vi "Get IC.vi"(8 "error in (no error)":errorcluster, 10 "Domain":refnum<class "NI_Domain.lvclass">, 11 "IC_2D_VIRef in":refnum<class "NI_IC_2D_VIRef.lvclass">) -> (0 "error out":errorcluster, 2 "IC":variant, 3 "IC_2D_VIRef out":refnum<class "NI_IC_2D_VIRef.lvclass">)   [LabVIEW 2020, in "NI_PDE.lvlib" / "NI_IC_2D_VIRef.lvclass"]
uses:
  <vilib>/gmath/pde.llb/ICClass/IC_2D_VIRef/NI_IC_2D_VIRef.lvclass
  <vilib>/gmath/pde.llb/DomainClass/NI_Domain.lvclass
  <vilib>/gmath/pde.llb/ICClass/IC_2D_VIRef/IC Data.ctl
  <vilib>/gmath/pde.llb/Common/PDE_IC Type.ctl
  <vilib>/gmath/pde.llb/ICClass/IC_2D_VIRef/NI_IC_2D_VIRef.lvclass/NI_IC_2D_VIRef.ctl
  <vilib>/gmath/NI_PDE.lvlib
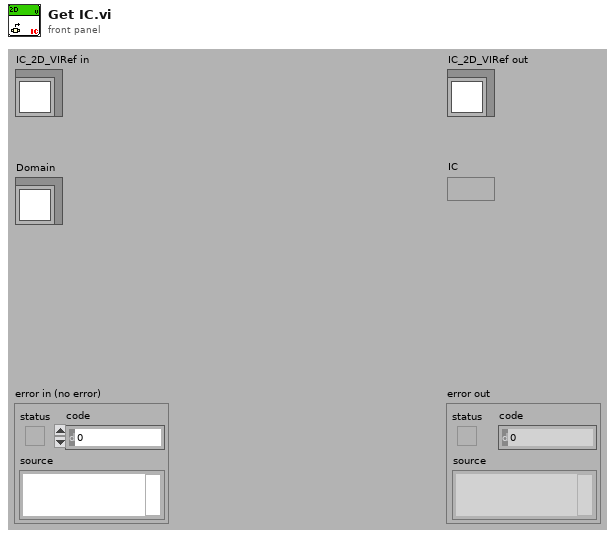
[diagram p1: front panel]
types:
  T1 = typedef "NI_PDE.lvlib/NI_IC_2D_VIRef.lvclass/IC Data.ctl" = cluster{"type":T2, "H":refnum<vi>, "data":variant}
  T2 = typedef "NI_PDE.lvlib/PDE_IC Type.ctl" = i32
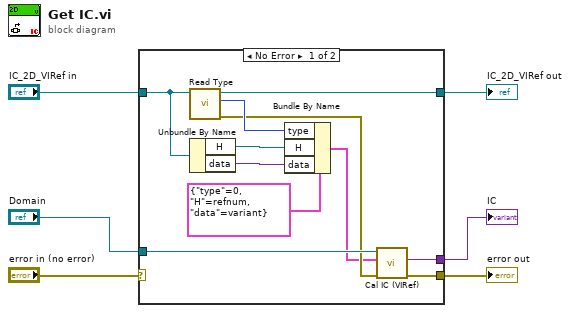
[diagram p0: block diagram]
diagram:
  n1 = case shown="No Error" "error in (no error)" {
    selector: "error in (no error)" -> [_ w19]
    tunnel: [w17 w18] -> w6
    tunnel: "IC_2D_VIRef in" -> [w14 w18]
    tunnel: "Domain" -> [w11 _]
    tunnel: [w7 w19] -> w3
    tunnel: [w8 _] -> w2
    frame No Error {
      n2 = call-dynamic "Read Type.vi"("IC.lvclass in"=w14) -> ("error out"=w10:errorcluster, "IC type"=w15:T2, "IC.lvclass out"=w17:refnum<class "NI_IC_2D_VIRef.lvclass">)  [unwired: 1 in, 7 out]
      n3 = Unbundle By Name(w14) -> ("H"=w13:refnum<vi>, "data"=w12:variant)
      n4 = Bundle By Name(cluster=T1 {"type"=0, "H"=refnum, "data"=variant} ("IC data"), "type"=w15, "H"=w13, "data"=w12) -> (w9:T1)
      n5 = call-dynamic "Cal IC (VIRef).vi"("error in (no error)"=w10, "IC in"=w9, "Domain in"=w11) -> ("error out"=w7:errorcluster, "IC out"=w8:variant)  [unwired: 7 out]
    }
    frame Error {
    }
  }
  "IC" <- w2
  "error out" <- w3
  "IC_2D_VIRef out" <- w6
